vi "SWERVE_DRIVE_MODULE_ACQUIRE.vi"(8 "Pass_Through_Time":dbl=-1.0 format="%33.4f", 11 "Swerve Module TypDef":T4) -> (0 "Swerve Rotational Speed":dbl, 1 "Swerve Rel Angle":dbl, 2 "Wheel Speed":dbl, 3 "Wheel Distance":dbl, 4 "Swerve Rel Rotation":T2 {"SIN" format="%13.4f"; "COS" format="%13.4f"; "VALUE" format="%13.4f"}, 5 "Swerve Module State":T3={"Speed"=0.0, "Angle"={"VALUE"=0.0, "COS"=1.0, "SIN"=0.0}} {"Angle"."SIN" format="%13.4f"; "Angle"."COS" format="%13.4f"; "Angle"."VALUE" format="%13.4f"}, 6 "SWERVE DRIVE MODULE POSITION":T1={"Distance"=0.0, "Angle"={"VALUE"=0.0, "COS"=1.0, "SIN"=0.0}, "P"=FALSE} {"Angle"."SIN" format="%13.4f"; "Angle"."COS" format="%13.4f"; "Angle"."VALUE" format="%13.4f"})   [LabVIEW 2019]
uses:
  <vilib>/Rock Robotics/WPI/ThirdParty/JAS_Junk/TrajLib/Trajectory_Library.lvlib
  <vilib>/Rock Robotics/SystemInterfaces/DIO/FPGA_DIOPWMChannel.ctl
  <vilib>/Rock Robotics/WPI/PWM/WPI_PWMDeadband.ctl
  <vilib>/Rock Robotics/WPI/MotorControl/WPI_MotorControlType.ctl
  <vilib>/Rock Robotics/SystemInterfaces/DIO/FPGA_DIOChannel.ctl
  <vilib>/Rock Robotics/WPI/MotorControl/WPI_MotorControlDeviceRef.ctl
  <vilib>/Rock Robotics/SystemInterfaces/Encoder/FPGA_EncoderIdx.ctl
  <vilib>/Rock Robotics/WPI/Encoder/WPI_EncoderType.ctl
  <vilib>/Rock Robotics/SystemInterfaces/Counter/FPGA_CounterCtrSystemIndex.ctl
  <vilib>/Rock Robotics/WPI/Encoder/WPI_EncoderDevRef.ctl
  SWERVE_DRIVE_MODULE_TYPDEF.ctl
  <vilib>/Rock Robotics/WPI/ThirdParty/JAS_Junk/TrajLib/TypeDef/ROTATION2D.ctl
  <vilib>/Rock Robotics/WPI/ThirdParty/JAS_Junk/TrajLib/TypeDef/SWERVE_DRIVE_MODULE_STATE.ctl
  <vilib>/Rock Robotics/WPI/ThirdParty/JAS_Junk/TrajLib/TypeDef/SWERVE_DRIVE_MODULE_POSITION.ctl
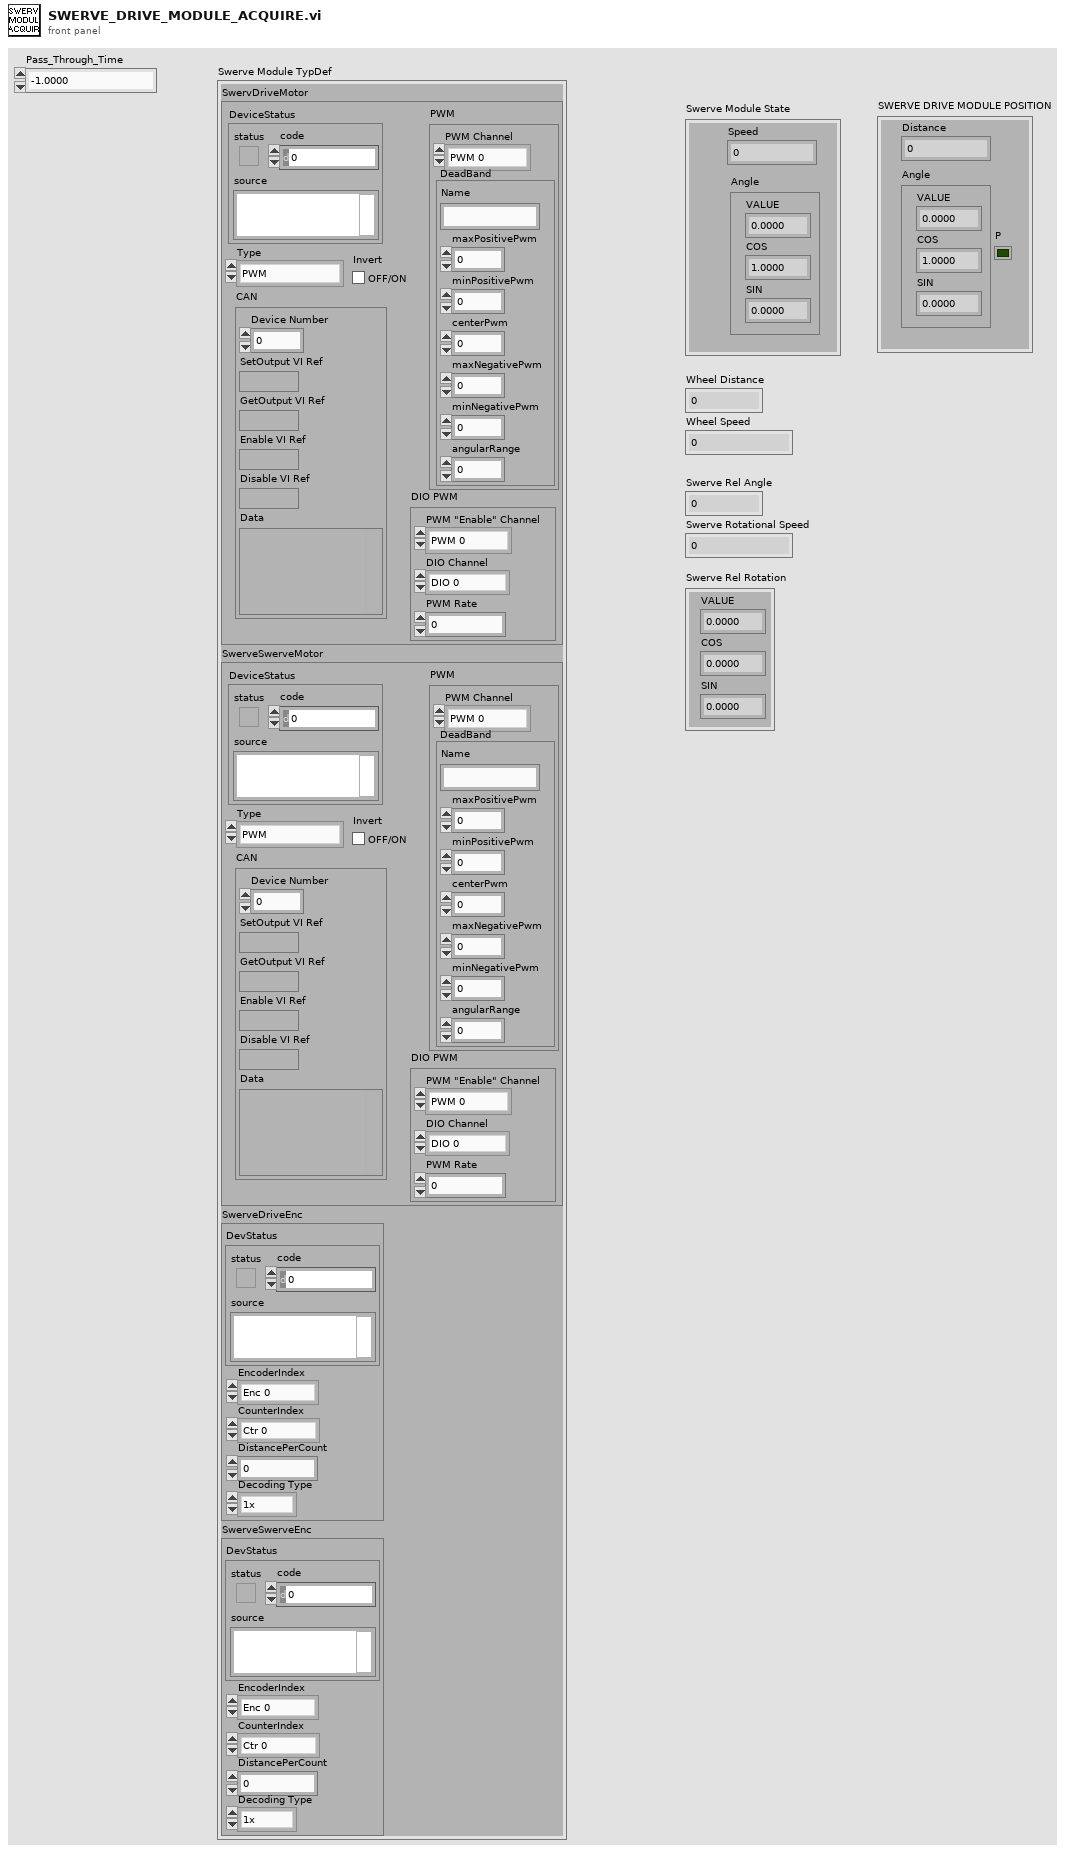
[diagram p1: front panel]
types:
  T1 = typedef "Trajectory_Library.lvlib/SWERVE_DRIVE_MODULE_POSITION.ctl" = cluster{"Distance":dbl, "Angle":T2, "P":bool}
  T2 = typedef "Trajectory_Library.lvlib/ROTATION2D.ctl" = cluster{"VALUE":dbl, "COS":dbl, "SIN":dbl}
  T3 = typedef "Trajectory_Library.lvlib/SWERVE_DRIVE_MODULE_STATE.ctl" = cluster{"Speed":dbl, "Angle":T2}
  T4 = typedef "SWERVE_DRIVE_MODULE_TYPDEF.ctl" = cluster{"SwervDriveMotor":T5, "SwerveSwerveMotor":T5, "SwerveDriveEnc":T10, "SwerveSwerveEnc":T10}
  T5 = typedef "WPI_MotorControlDeviceRef.ctl" = cluster{"DeviceStatus":errorcluster, "Type":T6, "PWM":cluster{"PWM Channel":T7, "DeadBand":T8}, "CAN":cluster{"Device Number":u8, "SetOutput VI Ref":variant, "GetOutput VI Ref":variant, "Enable VI Ref":variant, "Disable VI Ref":variant, "Data":variant}, "Invert":bool, "DIO PWM":cluster{"PWM \"Enable\" Channel":T7, "DIOChannel":T9, "PWM Rate":dbl}}
  T6 = typedef "WPI_MotorControlType.ctl" = enum16{"PWM", "CAN", "DIO PWM"}
  T7 = typedef "FPGA_DIOPWMChannel.ctl" = enum8{"PWM 0", "PWM 1", "PWM 2", "PWM 3", "PWM 4", "PWM 5", "PWM 6", "PWM 7", "PWM 8", "PWM 9", "PWM MXP 0", "PWM MXP 1", "PWM MXP 2", "PWM MXP 3", "PWM MXP 4", "PWM MXP 5", "PWM MXP 6", "PWM MXP 7", "PWM MXP 8", "PWM MXP 9", "Invalid"}
  T8 = typedef "WPI_PWMDeadband.ctl" = cluster{"Name":string, "maxPositivePwm":i32, "minPositivePwm":i32, "centerPwm":i32, "maxNegativePwm":i32, "minNegativePwm":i32, "angularRange":u16}
  T9 = typedef "FPGA_DIOChannel.ctl" = enum8{"DIO 0", "DIO 1", "DIO 2", "DIO 3", "DIO 4", "DIO 5", "DIO 6", "DIO 7", "DIO 8", "DIO 9", "DIO MXP 0", "DIO MXP 1", "DIO MXP 2", "DIO MXP 3", "DIO MXP 4", "DIO MXP 5", "DIO MXP 6", "DIO MXP 7", "DIO MXP 8", "DIO MXP 9", "DIO MXP 10", "DIO MXP 11", "DIO MXP 12", "DIO MXP 13", "DIO MXP 14", "DIO MXP 15", "SPI Port CS1", "SPI Port CS2", "SPI Port CS3", "SPI Port MISO", "SPI Port MOSI", "Invalid"}
  T10 = typedef "WPI_EncoderDevRef.ctl" = cluster{"DevStatus":errorcluster, "EncoderIndex":T11, "CounterIndex":T12, "DistancePerCount":dbl, "Decoding Type":T13}
  T11 = typedef "FPGA_EncoderIdx.ctl" = enum8{"Enc 0", "Enc 1", "Enc 2", "Enc 3", "Enc 4", "Enc 5", "Enc 6", "Enc 7", "Invalid"}
  T12 = typedef "FPGA_CounterCtrSystemIndex.ctl" = enum8{"Ctr 0", "Ctr 1", "Ctr 2", "Ctr 3", "Ctr 4", "Ctr 5", "Ctr 6", "Ctr 7", "Invalid"}
  T13 = typedef "WPI_EncoderType.ctl" = enum16{"1x", "2x", "4x"}
  T14 = typedef "SWERVE_MODULE_MOTOR_CO.ctl" = cluster{"WheelMotorDmd":dbl, "SwerveMotorDmd":dbl}
  T15 = typedef "SWERVE_MODULE_MOTOR_PV.ctl" = cluster{"WheelMotorSpd":dbl, "SwerveMotorSpd":dbl, "WheelDist":dbl, "SwerveAngle":dbl}
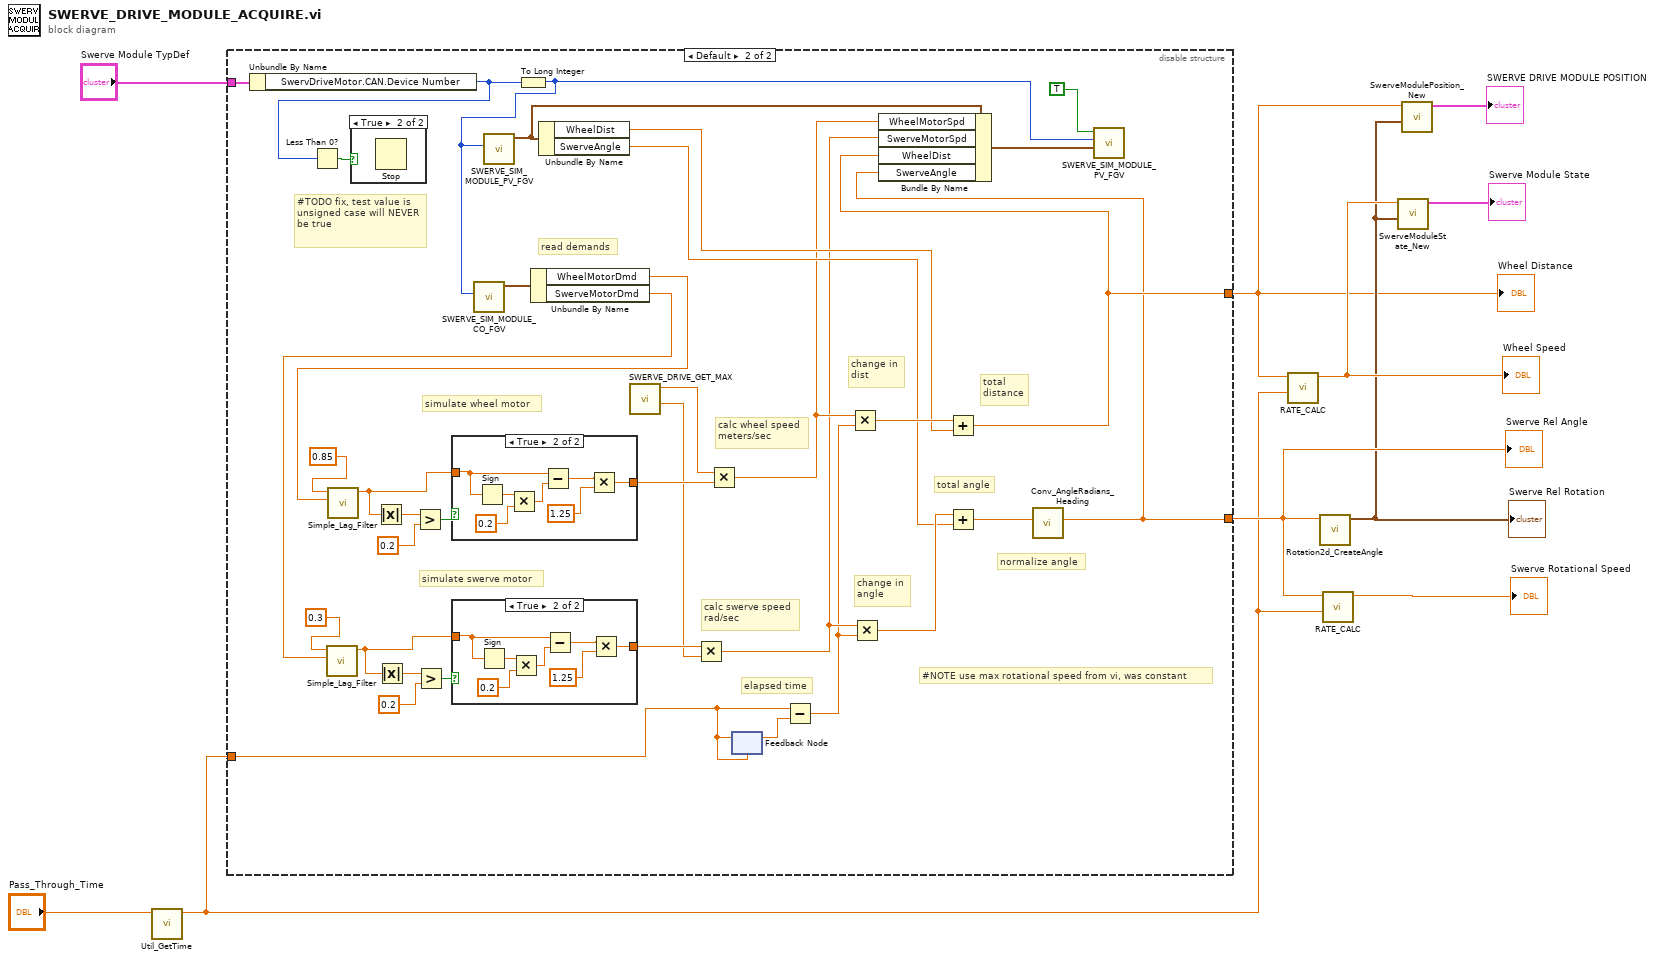
[diagram p0: block diagram]
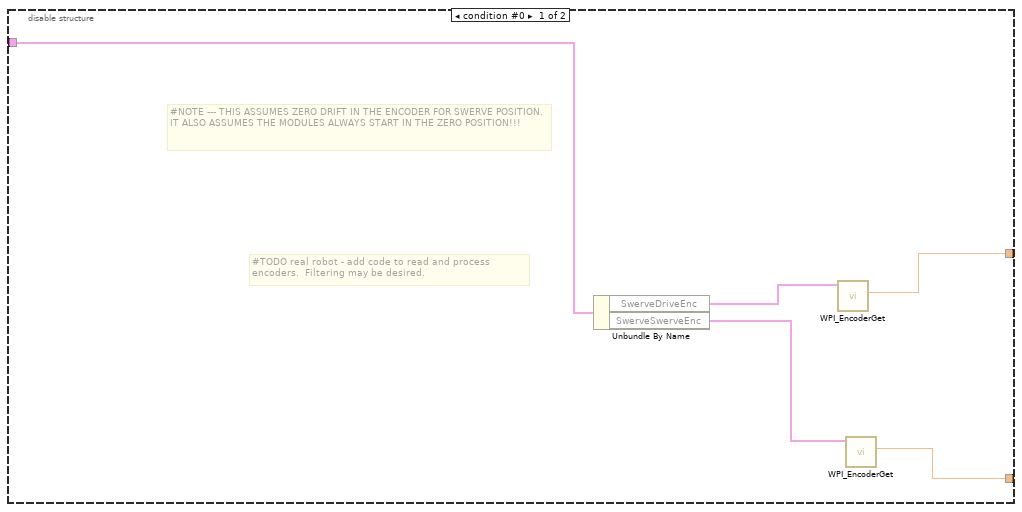
[diagram p2: hidden frame]
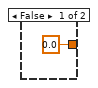
[diagram p3: hidden frame]
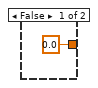
[diagram p4: hidden frame]
diagram:
  n1 = call <vilib>:"Util_GetTime.vi"("Pass_Through_Time"="Pass_Through_Time") -> ("FPGA_Time_Seconds"=w1:dbl)  [unwired: 9 in, 1 out]
  n2 = disable-structure shown="Default" {
    disable-tunnel: [w13 w43] -> w4
    disable-tunnel: [w12 w17] -> w6
    disable-tunnel: "Swerve Module TypDef" -> [w11 w51]
    disable-tunnel: w1 -> [_ w16]
    frame condition #0 {
      # "#TODO real robot - add code to read and process encoders.  Filtering may be desired."
      # "#NOTE --- THIS ASSUMES ZERO DRIFT IN THE ENCODER FOR SWERVE POSITION.  IT ALSO ASSUMES THE MODULES ALWAYS START IN THE ZERO POSITION!!!"
      n3 = Unbundle By Name(w11) -> ("SwerveDriveEnc"=w14:T10, "SwerveSwerveEnc"=w15:T10)
      n4 = call <vilib>:"WPI_EncoderGet.vi"("EncoderDevRef"=w14) -> ("Distance"=w13:dbl)  [unwired: 5 in, 5 out]
      n5 = call <vilib>:"WPI_EncoderGet.vi"("EncoderDevRef"=w15) -> ("Distance"=w12:dbl)  [unwired: 5 in, 5 out]
    }
    frame condition #1 (active) {
      # "normalize angle"
      # "total angle"
      # "total \ndistance"
      # "change in\nangle"
      # "change in\ndist"
      # "calc wheel speed\nmeters/sec"
      # "calc swerve speed\nrad/sec"
      # "simulate swerve motor"
      # "simulate wheel motor"
      # "#NOTE use max rotational speed from vi, was constant"
      # "#TODO fix, test value is unsigned case will NEVER be true"
      # "elapsed time"
      # "read demands"
      n6 = Unbundle By Name(w51) -> ("SwervDriveMotor.CAN.Device Number"=w22:u8)
      n7 = Less Than 0?(x=w22) -> (x < 0?=w39:bool)
      n8 = case shown="True" w39 {
        frame False {
        }
        frame True {
          n9 = Stop() -> ()  [unwired: 1 in]
        }
      }
      n10 = To Long Integer(number=w22) -> (32bit integer=w21:i32)
      n11 = call "SWERVE_SIM_MODULE_CO_FGV.vi"("Index"=w21) -> ("out SwerveModuleMotorDmd"=w42:T14)  [unwired: 10 in]
      n12 = call "SWERVE_SIM_MODULE_PV_FGV.vi"("Index"=w21) -> ("Out SwerveModulePV"=w41:T15)  [unwired: 10 in]
      n13 = Unbundle By Name(w42) -> ("WheelMotorDmd"=w28:dbl, "SwerveMotorDmd"=w35:dbl)
      n14 = call "Simple_Lag_Filter.vi"("Input"=w35, "Lag"=0.3) -> ("Lagged Ouptut"=w34:dbl)  [unwired: 9 in]
      n15 = call "Simple_Lag_Filter.vi"("Input"=w28, "Lag"=0.85) -> ("Lagged Ouptut"=w29:dbl)  [unwired: 9 in]
      n16 = Absolute Value(x=w29) -> (abs(x)=w32:dbl)
      n17 = Absolute Value(x=w34) -> (abs(x)=w38:dbl)
      n18 = Greater?(x=w32, y=0.2) -> (0:w30:bool)
      n19 = Greater?(x=w38, y=0.2) -> (0:w36:bool)
      n20 = case shown="True" w30 {
        tunnel: w29 -> [_ w57]
        tunnel: [0.0 w53] -> w27
        frame False {
        }
        frame True {
          n21 = Sign(1:w57) -> (0:w59:dbl)
          n22 = Multiply(x=w59, y=0.2) -> (x*y=w56:dbl)
          n23 = Subtract(x=w57, y=w56) -> (x-y=w55:dbl)
          n24 = Multiply(x=w55, y=1.25) -> (x*y=w53:dbl)
        }
      }
      n25 = case shown="True" w36 {
        tunnel: w34 -> [_ w65]
        tunnel: [0.0 w61] -> w33
        frame False {
        }
        frame True {
          n26 = Sign(1:w65) -> (0:w67:dbl)
          n27 = Multiply(x=w67, y=0.2) -> (x*y=w64:dbl)
          n28 = Subtract(x=w65, y=w64) -> (x-y=w63:dbl)
          n29 = Multiply(x=w63, y=1.25) -> (x*y=w61:dbl)
        }
      }
      n30 = Unbundle By Name(w41) -> ("WheelDist"=w47:dbl, "SwerveAngle"=w46:dbl)
      n31 = call "SWERVE_DRIVE_GET_MAX.vi"() -> ("Max Rotational Vel (Rad/Sec)"=w23:dbl, "Max Wheel Vel (Meter/Sec)"=w26:dbl)  [unwired: 10 in]
      n32 = Multiply(x=w33, y=w23) -> (x*y=w44:dbl)
      n33 = Multiply(x=w26, y=w27) -> (x*y=w45:dbl)
      n34 = feedback #1(w16) -> (w25:dbl)
      n35 = feedback-in #1(w16) -> ()
      n36 = Subtract(x=w16, y=w25) -> (x-y=w24:dbl)
      n37 = Multiply(x=w45, y=w24) -> (x*y=w49:dbl)
      n38 = Multiply(x=w44, y=w24) -> (x*y=w50:dbl)
      n39 = Add(x=w49, y=w47) -> (x+y=w43:dbl)
      n40 = Add(x=w50, y=w46) -> (x+y=w18:dbl)
      n41 = call <vilib>:"Conv_AngleRadians_Heading.vi"("Radians"=w18) -> ("Heading"=w17:dbl)  [unwired: 10 in]
      n42 = Bundle By Name(cluster=w41, "WheelMotorSpd"=w45, "SwerveMotorSpd"=w44, "WheelDist"=w43, "SwerveAngle"=w17) -> (w40:T15)
      n43 = call "SWERVE_SIM_MODULE_PV_FGV.vi"("In SwerveModulePV"=w40, "Index"=w21, "WRITE"=TRUE) -> ()  [unwired: 8 in, 1 out]
    }
  }
  "Wheel Distance" <- w4
  "Swerve Rel Angle" <- w6
  n44 = call "RATE_CALC.vi"("Time"=w1, "Input"=w4) -> ("Output"=w8:dbl)  [unwired: 9 in]
  "Wheel Speed" <- w8
  n45 = call <vilib>:"Rotation2d_CreateAngle.vi"("Angle"=w6) -> ("ROTATION"=w5:T2)  [unwired: 10 in]
  "Swerve Rel Rotation" <- w5
  n46 = call "RATE_CALC.vi"("Time"=w1, "Input"=w6) -> ("Output"=→"Swerve Rotational Speed":dbl)  [unwired: 9 in]
  n47 = call <vilib>:"SwerveModuleState_New.vi"("ROTATION"=w5, "Speed"=w8) -> ("SWERVE_DRIVE_MODULE_STATE"=→"Swerve Module State":T3)  [unwired: 9 in]
  n48 = call <vilib>:"SwerveModulePosition_New.vi"("ROTATION"=w5, "Distance"=w4) -> ("SWERVE_DRIVE_MODULE_POSITION"=→"SWERVE DRIVE MODULE POSITION":T1)  [unwired: 9 in]
